vi "PwrMeterSetup.vi"(0 "VISA IN":refnum<visa-resource-name>="GPIB1::16::INSTR", 2 "PwrMtrAdd":i32=13, 5 "error in":errorcluster, 7 "Channel":i32=1, 8 "Settling Tolerance(dB)":dbl=0.1, 10 "PwrMtr Readingds":i32=5) -> (14 "VISA Out":refnum<visa-resource-name>, 19 "error out":errorcluster)   [LabVIEW 2018, in "PNA-X.lvlib"]
doc: "' Set the number of sweep points to 21 on Channel 1.\n\nstatus = myGPIBWrite(viPNA, \"SENS1:SWE:POIN 21\")\n\nIf (status < VI_SUCCESS) Then HandleVISAError\n\n \n\n' Specify the GPIB address of the power meter\n\n' that will be used in performing the calibration.\n\nstatus = myGPIBWrite(viPNA, \"SYST:COMM:GPIB:PMET:ADDR 13\")\n\nIf (status < VI_SUCCESS) Then HandleVISAError\n\n \n\n' Turn use of the loss table OFF (this assumes there is\n\n' virtually no loss in the RF path to the power sensor\n\n' due to a splitter, coupler or adapter).\n\nstatus = myGPIBWrite(viPNA, \"SOUR:POW:CORR:COLL:TABL:LOSS OFF\")\n\nIf (status < VI_SUCCESS) Then HandleVISAError\n\n \n\n' Turn frequency checking OFF (so one power sensor is used for the entire cal\n\n' acquisition sweep regardless of frequency span).\n\nstatus = myGPIBWrite(viPNA, \"SOUR:POW:CORR:COLL:FCH OFF\")\n\nIf (status < VI_SUCCESS) Then HandleVISAError\n\n \n\n' Specify a nominal power accuracy tolerance (NTOLerance) in dB for the calibration,\n\n' and the maximum number (COUNt) of iterations to adjust power at each point,\n\n' attempting to achieve within tolerance of the desired power. If at any stimulus\n\n' point the power fails to reach within the set tolerance of the desired power\n\n' after the maximum number of iterations, the power at that point will be set to the\n\n' value determined by the last iteration (the Source Power Cal dialog box will\n\n' indicate the FAIL, but we can still apply the cal if desired when it's complete).\n\n' Each iteration is based upon a SETTLED power reading (see comments preceding the\n\n' next two commands below).\n\nstatus = myGPIBWrite(viPNA, \"SOUR1:POW2:CORR:COLL:ITER:NTOL 0.1\")\n\nIf (status < VI_SUCCESS) Then HandleVISAError\n\nstatus = myGPIBWrite(viPNA, \"SOUR1:POW2:CORR:COLL:ITER:COUN 3\")\n\nIf (status < VI_SUCCESS) Then HandleVISAError\n\n \n\n' The worst-case window of power uncertainty (for a calibration which meets\n\n' tolerance) is the sum of the iteration tolerance and the power meter settling\n\n' tolerance (which is described below).\n\n \n\n' At each stimulus point, the PNA takes power meter readings and determine when\n\n' they have settled by comparing the magnitude difference between consecutive\n\n' readings versus a nominal dB tolerance limit (NTOLerance) on that magnitude\n\n' difference. When consecutive readings are within tolerance of each other, or\n\n' if they are not within tolerance but we've taken a maximum number of readings\n\n' (COUNt), the PNA does a weighted average of the readings taken at that stimulus\n\n' point and that is considered our settled power reading.\n\nstatus = myGPIBWrite(viPNA, \"SOUR1:POW2:CORR:COLL:AVER:NTOL 0.1\")\n\nIf (status < VI_SUCCESS) Then HandleVISAError\n\nstatus = myGPIBWrite(viPNA, \"SOUR1:POW2:CORR:COLL:AVER:COUN 5\")\n\nIf (status < VI_SUCCESS) Then HandleVISAError\n\n \n\n' Specify if the cal power level is offset (positive value for a gain, negative\n\n' value for a loss) from the PNA port power setting on the channel when no source\n\n' power cal is active. This is to account for components between the PNA test\n\n' port and cal reference plane. In this example, we will calibrate at the PNA\n\n' test port, so there is no offset (it is zero).\n\n \n\nstatus = myGPIBWrite(viPNA, \"SOUR1:POW2:CORR:OFFS 0 DB\")\n\nIf (status < VI_SUCCESS) Then HandleVISAError\n\n \n\n' Show the source power cal dialog during the source power cal acquisition.\n\n' (this is the default, so this command is only necessary if this setting\n\n' may have been changed beforehand, perhaps by another program).\n\nstatus = myGPIBWrite(viPNA, \"SOUR1:POW2:CORR:COLL:DISP ON\")\n\nIf (status < VI_SUCCESS) Then HandleVISAError\n\n \n\n' Specify the method (type of device) that will be used to perform the cal.\n\n' Choose from power meter (PMETer), power meter and receiver (PMReceiver)\n\n' or just receiver (RECeiver).\n\n' PMReceiver uses the power meter for the first iteration of each point and\n\n' the PNA's reference receiver for subsequent iterations, so is much faster\n\n' than using power meter only. But the power meter accounts for compression\n\n' when calibrating at the output of an active device, whereas the reference\n\n' receiver cannot unless it is coupled to the cal reference plane (on a PNA\n\n' which allows direct access to the receivers).\n\n' Perform the source power cal acquisition sweep using the sensor attached to\n\n' Channel A of the power meter (asking for an OPC reply when it’s done). This\n\n' assumes that the power sensor is already connected to Port 2 of the PNA.\n\n \n\n' We'll put up an hourglass cursor while waiting for the acquire to complete.\n\nScreen.MousePointer = vbHourglass\n\nstatus = myGPIBWrite(viPNA, \"SOUR1:POW2:CORR:COLL:ACQ PMET,'ASEN';*OPC?\")\n\nIf (status < VI_SUCCESS) Then HandleVISAError\n\n' Other valid selections would be the following:\n\n‘ This mode uses Power Meter and Reference Receiver\n\n‘status = myGPIBWrite(viPNA, \"SOUR1:POW2:CORR:COLL:ACQ PMR,'BSEN';*OPC?\")\n\n‘ This mode uses PNA receiver only (no power meter)\n\n‘status = myGPIBWrite(viPNA, \"SOUR1:POW2:CORR:COLL:ACQ REC,'b1';*OPC?\")\n\n \n\n' In the process of beginning a source power cal acquisition, the PNA searches\n\n' for the power meter on VISA interfaces configured in the Agilent I/O Libraries\n\n' on the PNA. One of those interfaces is the SICL/VISA LAN server, so if this\n\n' program is using that interface, we need to ensure our program is not pending\n\n' an operation on that interface when the PNA wants to search it. So this\n\n' Wait subroutine suspends execution of our program (for 6000 milliseconds =\n\n' 6 seconds), giving the PNA time to search that interface and discover that the\n\n' power meter is not there (the 6 seconds is just to be safe, the search actually\n\n' takes only a few seconds).\n\n' Note: If instead of using the VISA LAN server interface, you are having this\n\n' program communicate with the PNA via it's GPIB interface (which requires the\n\n' power meter be connected to a different GPIB interface on the PNA, such as the\n\n' Agilent 82357A USB-to-GPIB), then this Wait is not needed.\n\nWait 6000\n\n \n\n' The PNA sends an OPC reply (\"+1\") when the cal acquisition is complete, so\n\n' our Read operation will wait on the reply until it is received. We need to\n\n' set the VISA timeout value long enough to give our Read sufficient time to\n\n' complete before a timeout error occurs. For this example, let's try setting\n\n' the limit to 60000 milliseconds (60 seconds).\n\nstatus = viSetAttribute(viPNA, VI_ATTR_TMO_VALUE, 60000)\n\nIf (status < VI_SUCCESS) Then HandleVISAError\n\nstatus = myGPIBRead(viPNA, strReply)\n\nIf (status < VI_SUCCESS) Then HandleVISAError\n\n \n\n' Change mouse cursor from hourglass back to normal\n\nScreen.MousePointer = vbDefault\n\n \n\n' Conclude the calibration. This applies the cal data to PNA channel memory,\n\n' and turns the correction ON for Port 2 on Channel 1,\n\n' but does NOT save the calibration.\n\nstatus = myGPIBWrite(viPNA, \"SOUR1:POW2:CORR:COLL:SAVE\")\n\nIf (status < VI_SUCCESS) Then HandleVISAError"
uses:
  PNA-X.lvlib
panel:
  in  "Power Meter Channel":string(combo)="A"
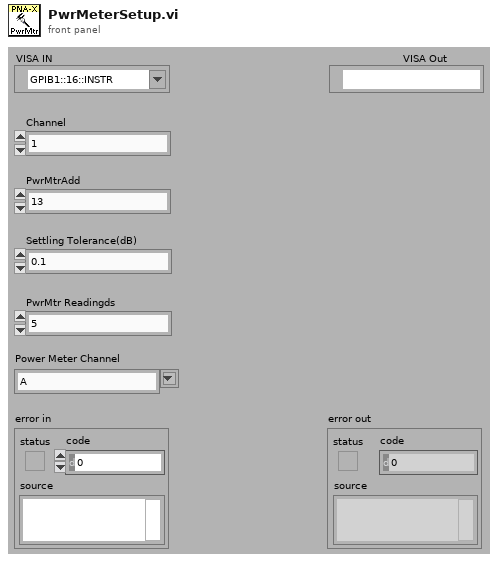
[diagram p1: front panel]
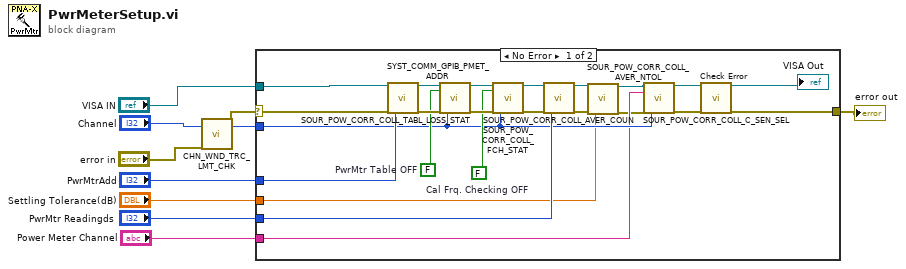
[diagram p0: block diagram]
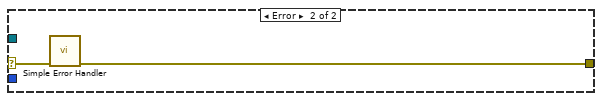
[diagram p2: hidden frame]
diagram:
  n1 = call "CHN_WND_TRC_LMT_CHK.vi"("Channel"="Channel", "error in"="error in") -> ("error out"=w6:errorcluster, "Channel"=w5:i32)  [unwired: 13 in, 3 out]
  n2 = case shown="No Error" w6 {
    selector: w6 -> [w25 w35]
    tunnel: [w22 w34] -> w4
    tunnel: "PwrMtrAdd" -> [w29 _]
    tunnel: "Settling Tolerance(dB)" -> [w13 _]
    tunnel: "PwrMtr Readingds" -> [w26 _]
    tunnel: w5 -> [w20 _]
    tunnel: "VISA IN" -> [w24 _]
    tunnel: "Power Meter Channel" -> [w18 _]
    frame No Error {
      w27 = FALSE  # Cal Frq. Checking OFF
      w28 = FALSE  # PwrMtr Table OFF
      n3 = call "SYST_COMM_GPIB_PMET_ADDR.vi"("VISA IN"=w24, "error in"=w25, "Address"=w29) -> ("VISA Out"=w32:refnum<visa-resource-name>, "error out"=w30:errorcluster)  [unwired: 15 in]
      n4 = call "SOUR_POW_CORR_COLL_TABL_LOSS_STAT.vi"("VISA IN"=w32, "Loss Table ON/OFF"=w28, "error in"=w30, "Channel"=w20) -> ("VISA Out"=w33:refnum<visa-resource-name>, "error out"=w31:errorcluster)  [unwired: 14 in]
      n5 = call "SOUR_POW_CORR_COLL_FCH_STAT.vi"("VISA IN"=w33, "Cal Frq. Checking ON/OFF"=w27, "error in"=w31, "Channel"=w20) -> ("VISA Out"=w12:refnum<visa-resource-name>, "error out"=w11:errorcluster)  [unwired: 14 in]
      n6 = call "SOUR_POW_CORR_COLL_AVER_COUN.vi"("VISA IN"=w12, "error in"=w11, "Max number of readings"=w26) -> ("VISA Out"=w16:refnum<visa-resource-name>, "error out"=w17:errorcluster)  [unwired: 15 in]
      n7 = call "SOUR_POW_CORR_COLL_AVER_NTOL.vi"("VISA IN"=w16, "error in"=w17, "Settling Tolerance(dB)"=w13) -> ("VISA Out"=w15:refnum<visa-resource-name>, "error out"=w14:errorcluster)  [unwired: 15 in]
      n8 = call "SOUR_POW_CORR_COLL_C_SEN_SEL.vi"("VISA IN"=w15, "Power Meter Channel"=w18, "error in"=w14, "Channel"=w20) -> ("VISA Out"=w19:refnum<visa-resource-name>, "error out"=w21:errorcluster)  [unwired: 14 in]
      n9 = call "Check Error.vi"("VISA Resource Name"=w19, "error in (no error)"=w21) -> ("dup VISA session"=→"VISA Out":refnum<visa-resource-name>, "error out"=w22:errorcluster)  [unwired: 16 in]
    }
    frame Error {
      n10 = call <vilib>:"Simple Error Handler.vi"("error in (no error)"=w35) -> ("error out"=w34:errorcluster)  [unwired: 4 in, 4 out]
    }
  }
  "error out" <- w4
